vi "Set Sample Rate.vi"(8 "error in (no error)":errorcluster, 10 "Sample Rate":u32, 11 "DeviceRefnum":u64) -> (0 "error out":errorcluster, 2 "function return":i32, 3 "DeviceRefnum Out":u64)   [LabVIEW 2014]
doc: "Set the sample rate for the device, also selects the baseband filters according to the requested sample rate for tuners where this is possible.\n Valid Ranges:\n 225001 - 300000 Hz\n 900001 - 3200000 Hz\n \nSample loss is to be expected for rates > 2400000"
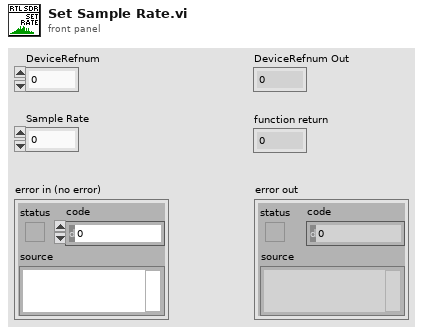
[diagram p1: front panel]
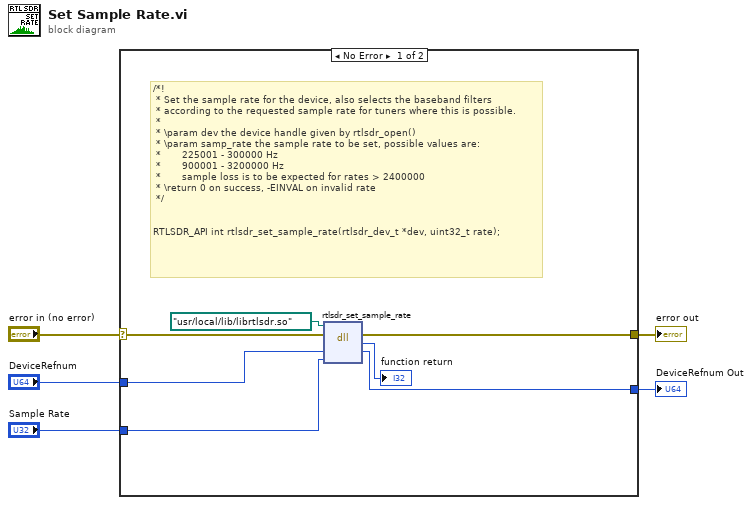
[diagram p0: block diagram]
diagram:
  n1 = case shown="No Error" "error in (no error)" {
    selector: "error in (no error)" -> [w6 w14]
    tunnel: "Sample Rate" -> [w11 _]
    tunnel: [w10 w14] -> w4
    tunnel: "DeviceRefnum" -> [w9 w13]
    tunnel: [w8 w13] -> w2
    frame No Error {
      # "/*!\n * Set the sample rate for the device, also selects the baseband filters\n * according to the requested sample rate for tuners where this is possible.\n *\n * \\param dev the device handle given by rtlsdr_open()\n * \\param samp_rate the sample rate to be set, possible values are:\n * \t\t    225001 - 300000 Hz\n * \t\t    900001 - 3200000 Hz\n * \t\t    sample loss is to be expected for rates > 2400000\n * \\return 0 on success, -EINVAL on invalid rate\n */\n\n\nRTLSDR_API int rtlsdr_set_sample_rate(rtlsdr_dev_t *dev, uint32_t rate);"
      n2 = dll-call lib="C:/Program Files (x86)/National Instruments/LabVIEW 2016/user.lib/rtlsdr/rtlsdr.*" fn="rtlsdr_set_sample_rate"(path in=path "/usr/local/lib/librtlsdr.so", error in=w6, "DeviceRefnum"=w9, "Sample Rate"=w11) -> (error out=w10:errorcluster, "return type"=→"function return":i32, "DeviceRefnum"=w8:u64)  [unwired: 2 in, 1 out]
    }
    frame Error {
    }
  }
  "error out" <- w4
  "DeviceRefnum Out" <- w2
